vi "测量流程.vi"(11 "控制命令":T1(ring)) -> ()   [LabVIEW 2016, in "斯坦道氟化物.lvlib"]
uses:
  <vilib>/ptbypt/NI_PtbyPt.lvlib
panel:
  out "start":timestamp
  out "重测":bool
  out "x-y":dbl
  out "当前时间":timestamp
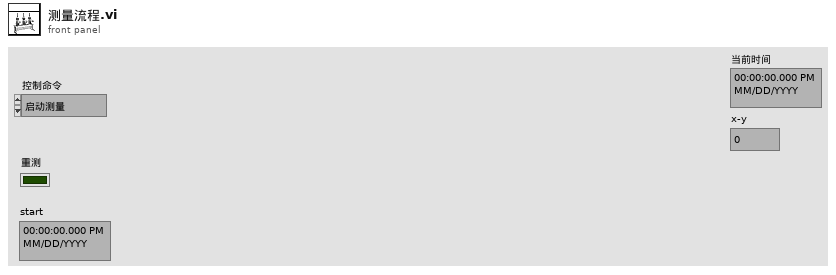
[diagram p1: front panel]
types:
  T1 = enum16{"启动测量", "标样核查", "零点核查", "跨度核查", "空白测试", "平行样测试", "加标回收", "空白校准", "标样校准", "初始化（清洗）", "停止测试", "仪器重启", "校时", "模式设置", "测量间隔设置"}
  T2 = cluster{"时间标识":timestamp, "设备":string, "日志信息":string, "流程参数":string}
  T3 = cluster{"站号":u16, "量程切换":enum32{"H", "L", "AUTO"}, "控制命令":enum16{"启动测量", "标样核查", "零点核查", "跨度核查", "空白测试", "平行样测试", "加标回收", "空白校准", "标样校准", "初始化（清洗）", "停止测试", "仪器重启", "校时", "模式设置", "测量间隔设置"}, "模式设置":enum16{"待机", "连续模式", "周期模式", "定点模式", "受控模式", "手动模式"}, "测量间隔":u16}
  T4 = typedef "报警信息字段定义.ctl" = cluster{"时间":timestamp, "参数":string, "报警信息":string, "备注":string, "code":u64}
  T5 = enum16{"空闲", "水样测试", "标样核查", "零点核查", "跨度核查", "空白测试", "平行样测试", "加标回收", "空白校准", "标样校准", "初始化（清洗）"}
  T6 = cluster{"因子编码":u32, "单位":u16, "标样参考值":sgl, "水样数据时间":timestamp, "水样实测值":sgl, "水样数据标识":string, "标样数据时间":timestamp, "标样实测值":sgl, "标样数据标识":string, "空白数据时间":timestamp, "空白实测值":sgl, "空白数据标识":string, "零点核查数据时间":timestamp, "零点核查实测值":sgl, "零点核查数据标识":string, "跨度核查数据时间":timestamp, "跨度核查实测值":sgl, "跨度核查数据标识":string, "加标回收数据时间":timestamp, "加标回收实测值":sgl, "加标回收数据标识":string, "平行样数据时间":timestamp, "平行样实测值":sgl, "平行样数据标识":string, "F0":sgl, "F1":sgl, "F2":sgl, "F3":sgl, "F4":sgl, "F5":sgl, "F6":sgl, "F7":sgl, "温度":sgl, "湿度":sgl, "X值":sgl, "fidrange":u16, "X1值":sgl}[]
  T7 = cluster{"因子编码":u32, "单位":u16, "标样参考值":sgl, "水样数据时间":timestamp, "水样实测值":sgl, "水样数据标识":string, "标样数据时间":timestamp, "标样实测值":sgl, "标样数据标识":string, "空白数据时间":timestamp, "空白实测值":sgl, "空白数据标识":string, "零点核查数据时间":timestamp, "零点核查实测值":sgl, "零点核查数据标识":string, "跨度核查数据时间":timestamp, "跨度核查实测值":sgl, "跨度核查数据标识":string, "加标回收数据时间":timestamp, "加标回收实测值":sgl, "加标回收数据标识":string, "平行样数据时间":timestamp, "平行样实测值":sgl, "平行样数据标识":string, "F0":sgl, "F1":sgl, "F2":sgl, "F3":sgl, "F4":sgl, "F5":sgl, "F6":sgl, "F7":sgl, "温度":sgl, "湿度":sgl, "X值":sgl, "fidrange":u16, "X1值":sgl}
  T8 = cluster{"总磷跨度值":dbl, "总磷零点标准液浓度":dbl, "总磷跨度标准液浓度":dbl, "总磷标准液标准浓度":dbl, "总氮跨度值":dbl, "总氮零点标准液浓度":dbl, "总氮跨度标准液浓度":dbl, "总氮标准液标准浓度":dbl, "COD跨度值":dbl, "COD零点标准液浓度":dbl, "COD跨度标准液浓度":dbl, "COD标准液标准浓度":dbl, "氨氮跨度值":dbl, "氨氮零点标准液浓度":dbl, "氨氮跨度标准液浓度":dbl, "氨氮标准液标准浓度":dbl, "磷酸盐跨度值":dbl, "磷酸盐零点标准液浓度":dbl, "磷酸盐跨度标准液浓度":dbl, "磷酸盐标准液标准浓度":dbl, "硝氮跨度值":dbl, "硝氮零点标准液浓度":dbl, "硝氮跨度标准液浓度":dbl, "硝氮标准液标准浓度":dbl, "亚硝氮跨度值":dbl, "亚硝氮零点标准液浓度":dbl, "亚硝氮跨度标准液浓度":dbl, "亚硝氮标准液标准浓度":dbl, "硫化物跨度值":dbl, "硫化物零点标准液浓度":dbl, "硫化物跨度标准液浓度":dbl, "硫化物标准液标准浓度":dbl, "硅酸盐跨度值":dbl, "硅酸盐零点标准液浓度":dbl, "硅酸盐跨度标准液浓度":dbl, "硅酸盐标准液标准浓度":dbl, "总磷零点标准液偏差":dbl, "总磷跨度标准液偏差":dbl, "总磷标准液标准偏差":dbl, "总氮零点标准液偏差":dbl, "总氮跨度标准液偏差":dbl, "总氮标准液标准偏差":dbl, "COD零点标准液偏差":dbl, "COD跨度标准液偏差":dbl, "COD标准液标准偏差":dbl, "氨氮零点标准液偏差":dbl, "氨氮跨度标准液偏差":dbl, "氨氮标准液标准偏差":dbl, "磷酸盐零点标准液偏差":dbl, "磷酸盐跨度标准液偏差":dbl, "磷酸盐标准液标准偏差":dbl, "硝氮零点标准液偏差":dbl, "硝氮跨度标准液偏差":dbl, "硝氮标准液标准偏差":dbl, "亚硝氮零点标准液偏差":dbl, "亚硝氮跨度标准液偏差":dbl, "亚硝氮标准液标准偏差":dbl, "硫化物零点标准液偏差":dbl, "硫化物跨度标准液偏差":dbl, "硫化物标准液标准偏差":dbl, "硅酸盐零点标准液偏差":dbl, "硅酸盐跨度标准液偏差":dbl, "硅酸盐标准液标准偏差":dbl, "氟化物跨度值":dbl, "氟化物零点标准液浓度":dbl, "氟化物跨度标准液浓度":dbl, "氟化物标准液标准浓度":dbl, "氟化物零点标准液偏差":dbl, "氟化物跨度标准液偏差":dbl, "氟化物标准液标准偏差":dbl}
  T9 = cluster{"系统时间":timestamp, "工作状态":u16, "测量模式":enum16{"待机", "连续模式", "周期模式", "定点模式", "受控模式", "手动模式"}, "告警代码":u16, "故障代码":u16, "日志代码":u16, "软件版本":u16, "F0":sgl, "F1":sgl, "F2":sgl, "F3":sgl, "T":sgl, "H":sgl, "id":u16, "flowid":u16, "量程":u16, "总磷控温温度1":sgl, "营养盐控温温度2":sgl, "ADC":sgl}
  T10 = cluster{"水样测试量程模式":enum16{"H", "L", "AUTO"}, "空白核查量程模式":enum16{"H", "L", "AUTO"}, "跨度核查量程模式":enum16{"H", "L", "AUTO"}, "加标回收量程模式":enum16{"H", "L", "AUTO"}, "标样核查量程模式":enum16{"H", "L", "AUTO"}}
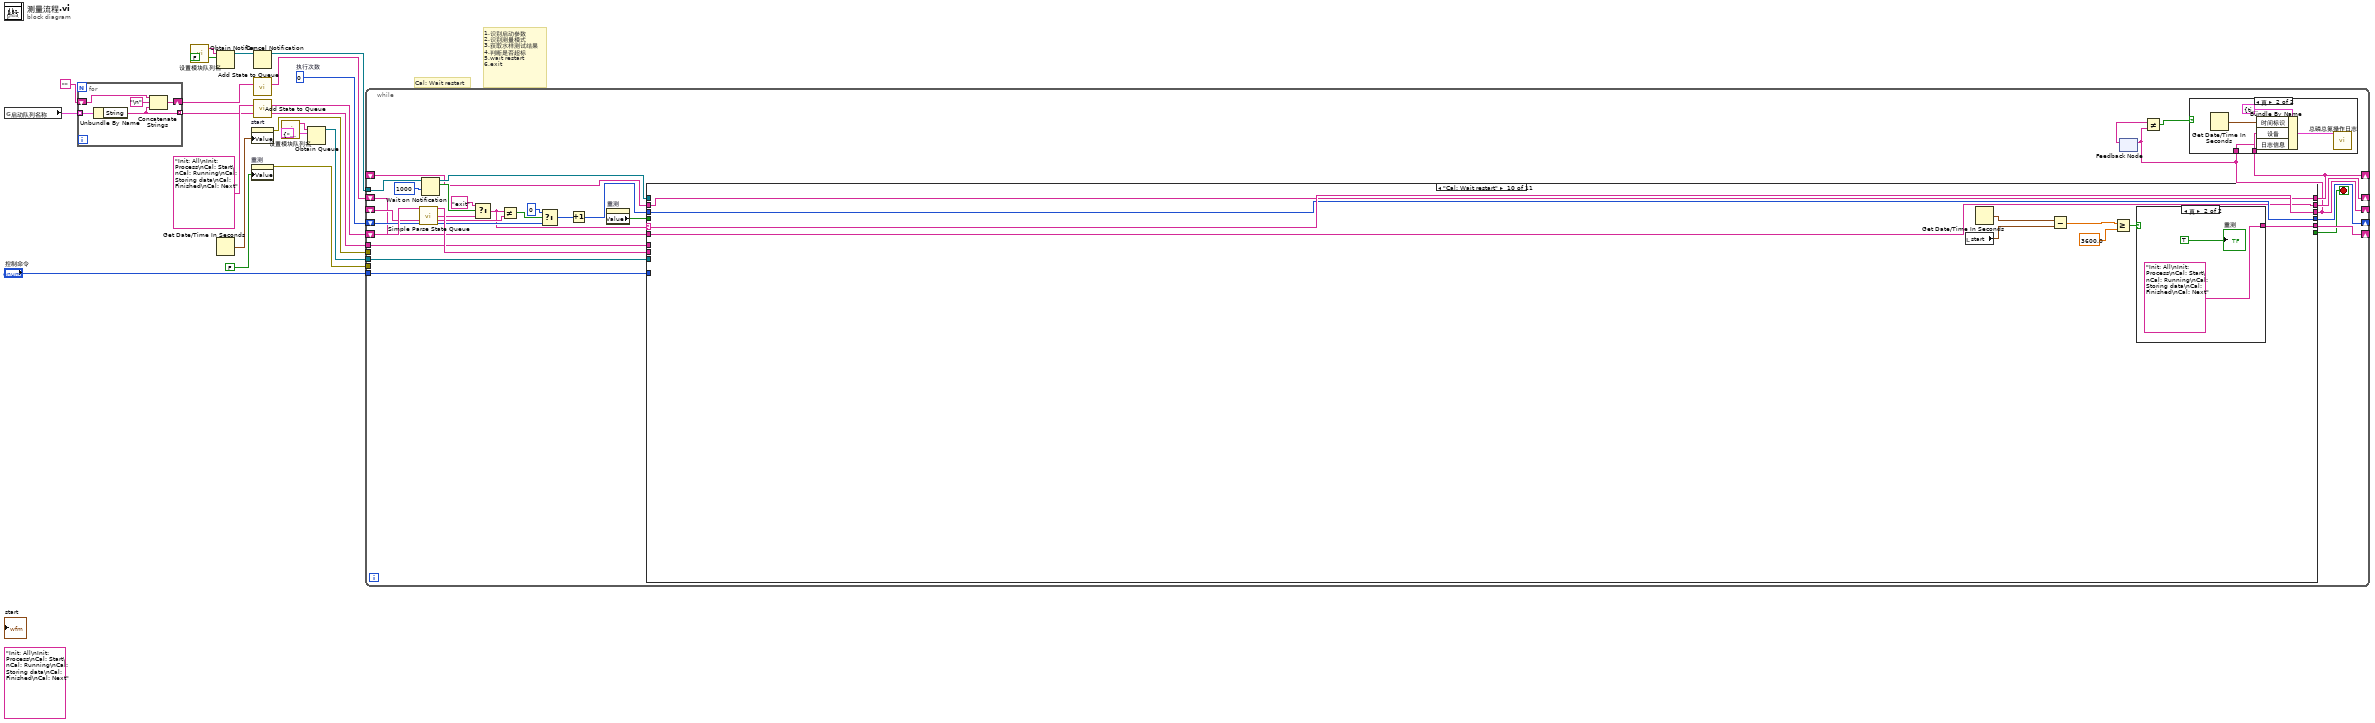
[diagram p0: block diagram]
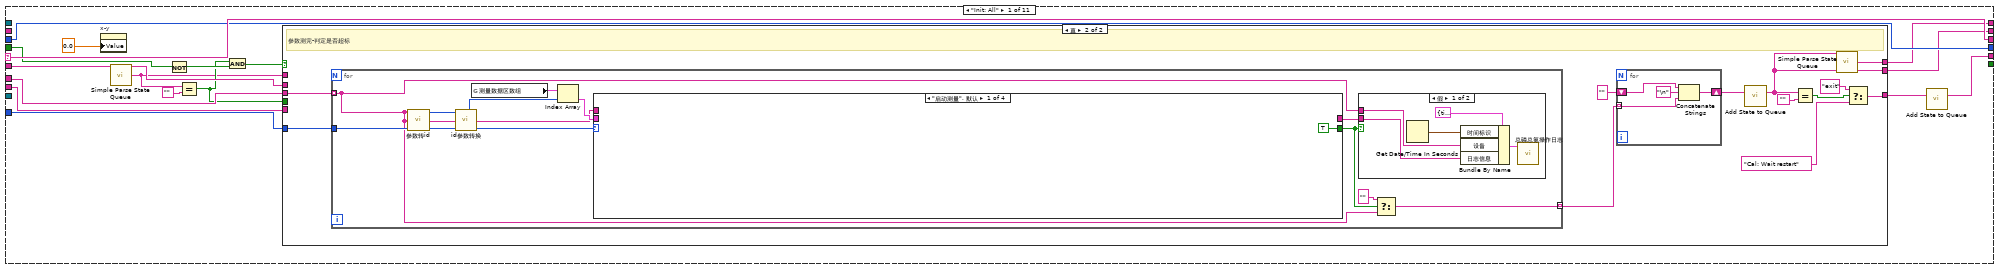
[diagram p3: hidden frame]
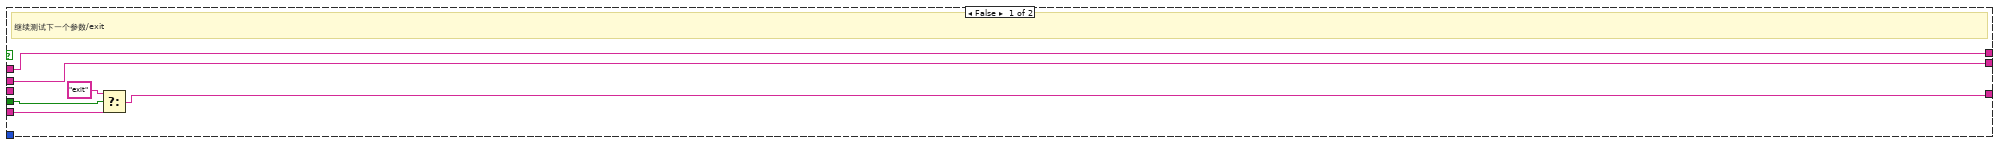
[diagram p4: hidden frame]
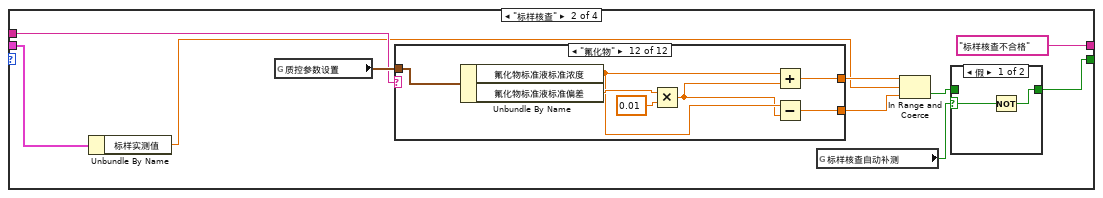
[diagram p6: hidden frame]
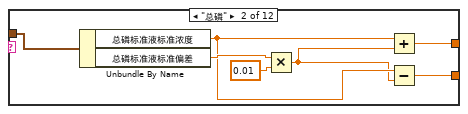
[diagram p9: hidden frame]
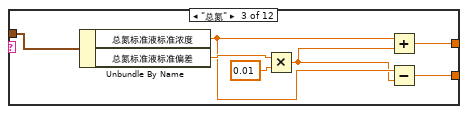
[diagram p10: hidden frame]
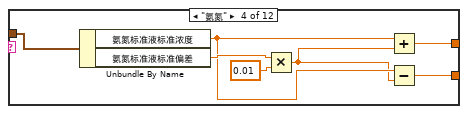
[diagram p11: hidden frame]
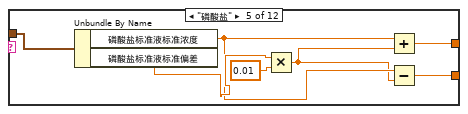
[diagram p12: hidden frame]
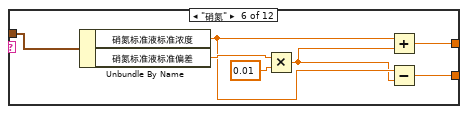
[diagram p13: hidden frame]
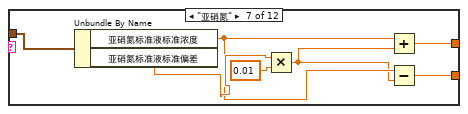
[diagram p14: hidden frame]
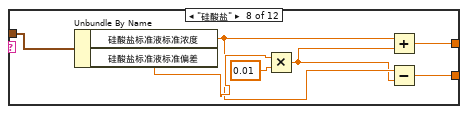
[diagram p15: hidden frame]
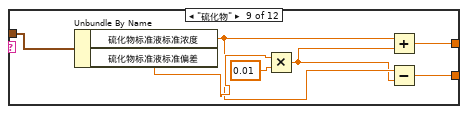
[diagram p16: hidden frame]
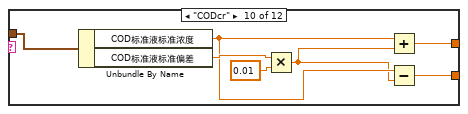
[diagram p17: hidden frame]
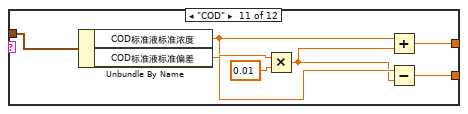
[diagram p18: hidden frame]
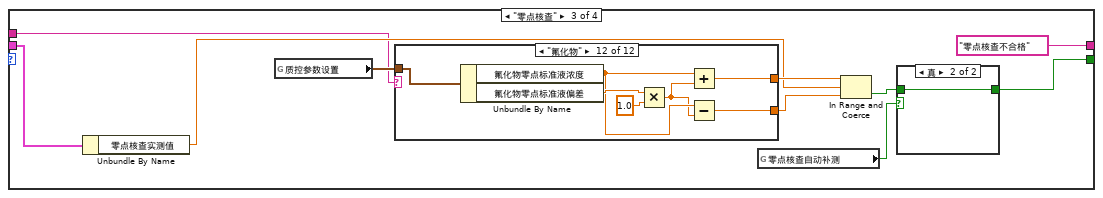
[diagram p19: hidden frame]
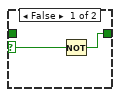
[diagram p20: hidden frame]
diagram:
  (unwired) "Init: All\nInit: Process\nCal: Start\nCal: Running\nCal: Storing data\nCal: Finished\nCal: Next" ("State(s) In (\"\")")
  w14 = 0  # 执行次数
  # "Cal: Wait restart"
  # "1.识别启动参数\n2.识别测量模式\n3.获取水样测试结果\n4.判断是否超标\n5.wait restart\n6.exit"
  n1 = global read "model config var.vi" "启动队列名称"() -> (w7:cluster{"String":string, "Value":u16}[])
  n2 = for {
    shift-right: [w24] -> w8
    shift-left: "" -> [w25]
    tunnel: w7 -> [w23] mode=indexing
    tunnel: [w21] -> w5 mode=indexing
    n3 = Unbundle By Name(w23) -> ("String"=w21:string)
    n4 = Concatenate Strings(w25, "\n", w21) -> (w24:string)
  }
  n5 = call "设置模块队列名.vi"() -> ("Msg"=w12:string)  [unwired: 5 in]
  n6 = Obtain Notifier(name (unnamed)=w12, notification data type=FALSE) -> (notifier out=w19:refnum<notifier>)  [unwired: 2 in, 2 out]
  n7 = Get Date/Time In Seconds() -> (seconds since 1Jan1904=w1:timestamp)
  n8 = property on="start" class="AbsTime (严格)"("Value"=w1) -> (error out=w2:errorcluster)  [unwired: 2 in, 1 out]
  n9 = property on="重测" class="Bool (严格)"("Value"=FALSE ("重测")) -> (error out=w3:errorcluster)  [unwired: 2 in, 1 out]
  n10 = Cancel Notification(0:w19) -> (8:w10:refnum<notifier>)  [unwired: 1 in, 2 out]
  n11 = call "Add State to Queue.vi"("State(s) In (\"\")"=w8) -> ("States Out"=w13:string)  [unwired: 14 in]
  n12 = call "Add State to Queue.vi"("State(s) In (\"\")"="Init: All\nInit: Process\nCal: Start\nCal: Running\nCal: Storing data\nCal: Finished\nCal: Next" ("State(s) In (\"\")")) -> ("States Out"=w17:string)  [unwired: 14 in]
  n13 = call "设置模块队列名.vi"() -> ("Msg"=w11:string)  [unwired: 5 in]
  n14 = Obtain Queue(name (unnamed)=w11, element data type=cluster{"命令":string, "data":variant} {"命令"="", "data"=variant}) -> (queue out=w15:refnum<queue>)  [unwired: 3 in, 2 out]
  n15 = while {
    tunnel: w15 -> [w52]
    shift-right: [w51] -> _
    shift-left: w17 -> [w54]
    shift-right: [w45] -> _
    shift-left: w14 -> [w48]
    shift-right: [w27] -> _
    shift-left: _ -> [w50]
    tunnel: "控制命令" -> [w43]
    shift-right: [w41] -> _
    shift-left: w13 -> [w31]
    shift-right: [w29] -> _
    shift-left: _ -> [w30]
    tunnel: w10 -> [w39]
    tunnel: w5 -> [w33]
    tunnel: w3 -> [_]
    tunnel: w2 -> [_]
    stop <- w42 stop-if-true
    n16 = call "Simple Parse State Queue.vi"("State Queue"=w54) -> ("Remain States"=w53:string, "Next State"=w36:string)  [unwired: 13 in]
    n17 = Wait on Notification(notifier=w39, timeout in ms (-1)=1000 ("超时毫秒(-1)")) -> (notifier out=w34:refnum<notifier>, notification=w38:bool)  [unwired: 2 in, 2 out]
    n18 = Select(t="exit", s=w38, f=w36) -> (s? t:f=w35:string)
    n19 = Not Equal?(x=w35, y=w50) -> (x != y?=w49:bool)
    n20 = Select(t=0, s=w49, f=w48) -> (s? t:f=w46:i32)
    n21 = Increment(x=w46) -> (x+1=w44:i32)
    n22 = property on="重测" class="Bool (严格)"() -> ("Value"=w32:bool)  [unwired: 2 in, 2 out]
    n23 = case shown="\"Cal: Wait restart\"" w35 {
      selector: w35 -> [w76 w394 w434 w495 w510 w516 w530 w547 w561 w572 w585]
      tunnel: w53 -> [w70 w404 w436 w497 _ w527 w535 w549 _ _ w586]
      tunnel: w52 -> [_ _ w432 _ _ _ _ _ _ _ w582]
      tunnel: [w77 w405 w435 w496 w511 w526 w534 w548 "Init: All\nInit: Process\nCal: Start\nCal: Running\nCal: Storing data\nCal: Finished\nCal: Next" ("State(s) In (\"\")") w567 w586] -> w51
      tunnel: [w76 w394 w434 w495 w510 w516 w530 w547 w561 w572 w585] -> w27
      tunnel: [w75 w393 w414 w494 w509 w519 w533 w545 w560 w571 w584] -> w45
      tunnel: w44 -> [w75 w393 w414 w494 w509 w519 w533 w545 w560 w571 w584]
      tunnel: w43 -> [w71 w398 w431 _ _ _ _ _ _ _ _]
      tunnel: [_ _ _ _ _ _ _ _ _ _ TRUE] -> w42
      tunnel: w31 -> [w68 w403 w422 w493 w503 w513 w537 w546 w559 w570 w583]
      tunnel: [w62 w401 w416 w492 w502 w512 w536 w544 w558 w569 w577] -> w29
      tunnel: [w66 w403 w422 w493 w503 w513 w537 w546 w559 w570 w583] -> w41
      tunnel: w30 -> [_ w401 w416 w492 w502 w512 w536 w544 w558 w569 w577]
      tunnel: w34 -> [_ _ _ _ _ _ _ _ _ _ w581]
      tunnel: w33 -> [w72 _ _ _ _ _ _ _ _ _ _]
      tunnel: w32 -> [w60 _ w413 _ _ _ _ w543 _ _ _]
      frame "Init: All" {
        n24 = property on="x-y" class="DigNum (严格)"("Value"=0.0 ("x-y")) -> ()  [unwired: 2 in, 2 out]
        n25 = call "Simple Parse State Queue.vi"("State Queue"=w68) -> ("Remain States"=w67:string, "Next State"=w61:string)  [unwired: 13 in]
        n26 = Not(x=w60) -> (.not. x?=w64:bool)
        n27 = Equal?(x=w61, y="") -> (x = y?=w63:bool)
        n28 = And(x=w63, y=w64) -> (x .and. y?=w65:bool)
        n29 = case shown="真" w65 {
          tunnel: w72 -> [_ w95]
          tunnel: w71 -> [_ w94]
          tunnel: w70 -> [w80 _]
          tunnel: [w79 w88] -> w69
          tunnel: w67 -> [w83 _]
          tunnel: [w83 w84] -> w66
          tunnel: w63 -> [w81 _]
          tunnel: [w78 w85] -> w62
          tunnel: w61 -> [w78 _]
          frame False {
            # "继续测试下一个参数/exit"
            n30 = Select(t="exit", s=w81, f=w80) -> (s? t:f=w79:string)
          }
          frame True {
            # "参数测完-判定是否超标"
            n31 = for {
              tunnel: w95 -> [w101] mode=indexing
              tunnel: w94 -> [w109]
              tunnel: [w103] -> w93 mode=indexing
              n32 = call "参数转id.vi"("table"=w101) -> ("id"=w108:u16)  [unwired: 10 in]
              n33 = call "id参数转换.vi"("id"=w108) -> ("数组资源索引"=w107:i32)  [unwired: 9 in, 1 out]
              n34 = global read "VAR总磷总氮全局变量.vi" "测量数据区数组"() -> (w106:T6)
              n35 = Index Array(array=w106, index=w107) -> (element=w105:T7)
              n36 = case shown="\"启动测量\", 默认" w109 {
                tunnel: w105 -> [_ w125 w210 w301]
                tunnel: w101 -> [_ w121 w211 w300]
                tunnel: [TRUE w116 w206 w296] -> w102
                tunnel: [_ "标样核查不合格" ("日志信息") "零点核查不合格" ("日志信息") "跨度核查不合格" ("日志信息")] -> w100
                frame "启动测量", Default {
                }
                frame "标样核查" {
                  n37 = Unbundle By Name(w125) -> ("标样实测值"=w120:sgl)
                  n38 = global read "总磷总氮断电保存全局变量.vi" "质控参数设置"() -> (w124:T8)
                  n39 = case shown="\"氟化物\"" w121 {
                    tunnel: w124 -> [_ w135 w138 w145 w152 w159 w166 w173 w180 w187 w194 w201]
                    tunnel: [_ w132 w137 w144 w151 w158 w165 w172 w179 w186 w193 w200] -> w123
                    tunnel: [_ w131 w136 w143 w150 w157 w164 w171 w178 w185 w192 w199] -> w122
                    frame Default {
                    }
                    frame "总磷" {
                      n40 = Unbundle By Name(w135) -> ("总磷标准液标准浓度"=w130:dbl, "总磷标准液标准偏差"=w134:dbl)
                      n41 = Multiply(x=w134, y=0.01) -> (x*y=w129:dbl)
                      n42 = Add(x=w130, y=w129) -> (x+y=w132:dbl)
                      n43 = Subtract(x=w130, y=w129) -> (x-y=w131:dbl)
                    }
                    frame "总氮" {
                      n44 = Unbundle By Name(w138) -> ("总氮标准液标准浓度"=w140:dbl, "总氮标准液标准偏差"=w142:dbl)
                      n45 = Multiply(x=w142, y=0.01) -> (x*y=w139:dbl)
                      n46 = Add(x=w140, y=w139) -> (x+y=w137:dbl)
                      n47 = Subtract(x=w140, y=w139) -> (x-y=w136:dbl)
                    }
                    frame "氨氮" {
                      n48 = Unbundle By Name(w145) -> ("氨氮标准液标准浓度"=w147:dbl, "氨氮标准液标准偏差"=w149:dbl)
                      n49 = Multiply(x=w149, y=0.01) -> (x*y=w146:dbl)
                      n50 = Add(x=w147, y=w146) -> (x+y=w144:dbl)
                      n51 = Subtract(x=w147, y=w146) -> (x-y=w143:dbl)
                    }
                    frame "磷酸盐" {
                      n52 = Unbundle By Name(w152) -> ("磷酸盐标准液标准浓度"=w154:dbl, "磷酸盐标准液标准偏差"=w156:dbl)
                      n53 = Multiply(x=w156, y=0.01) -> (x*y=w153:dbl)
                      n54 = Add(x=w154, y=w153) -> (x+y=w151:dbl)
                      n55 = Subtract(x=w154, y=w153) -> (x-y=w150:dbl)
                    }
                    frame "硝氮" {
                      n56 = Unbundle By Name(w159) -> ("硝氮标准液标准浓度"=w161:dbl, "硝氮标准液标准偏差"=w163:dbl)
                      n57 = Multiply(x=w163, y=0.01) -> (x*y=w160:dbl)
                      n58 = Add(x=w161, y=w160) -> (x+y=w158:dbl)
                      n59 = Subtract(x=w161, y=w160) -> (x-y=w157:dbl)
                    }
                    frame "亚硝氮" {
                      n60 = Unbundle By Name(w166) -> ("亚硝氮标准液标准浓度"=w168:dbl, "亚硝氮标准液标准偏差"=w170:dbl)
                      n61 = Multiply(x=w170, y=0.01) -> (x*y=w167:dbl)
                      n62 = Add(x=w168, y=w167) -> (x+y=w165:dbl)
                      n63 = Subtract(x=w168, y=w167) -> (x-y=w164:dbl)
                    }
                    frame "硅酸盐" {
                      n64 = Unbundle By Name(w173) -> ("硅酸盐标准液标准浓度"=w175:dbl, "硅酸盐标准液标准偏差"=w177:dbl)
                      n65 = Multiply(x=w177, y=0.01) -> (x*y=w174:dbl)
                      n66 = Add(x=w175, y=w174) -> (x+y=w172:dbl)
                      n67 = Subtract(x=w175, y=w174) -> (x-y=w171:dbl)
                    }
                    frame "硫化物" {
                      n68 = Unbundle By Name(w180) -> ("硫化物标准液标准浓度"=w182:dbl, "硫化物标准液标准偏差"=w184:dbl)
                      n69 = Multiply(x=w184, y=0.01) -> (x*y=w181:dbl)
                      n70 = Add(x=w182, y=w181) -> (x+y=w179:dbl)
                      n71 = Subtract(x=w182, y=w181) -> (x-y=w178:dbl)
                    }
                    frame "CODcr" {
                      n72 = Unbundle By Name(w187) -> ("COD标准液标准浓度"=w189:dbl, "COD标准液标准偏差"=w191:dbl)
                      n73 = Multiply(x=w191, y=0.01) -> (x*y=w188:dbl)
                      n74 = Add(x=w189, y=w188) -> (x+y=w186:dbl)
                      n75 = Subtract(x=w189, y=w188) -> (x-y=w185:dbl)
                    }
                    frame "COD" {
                      n76 = Unbundle By Name(w194) -> ("COD标准液标准浓度"=w196:dbl, "COD标准液标准偏差"=w198:dbl)
                      n77 = Multiply(x=w198, y=0.01) -> (x*y=w195:dbl)
                      n78 = Add(x=w196, y=w195) -> (x+y=w193:dbl)
                      n79 = Subtract(x=w196, y=w195) -> (x-y=w192:dbl)
                    }
                    frame "氟化物" {
                      n80 = Unbundle By Name(w201) -> ("氟化物标准液标准浓度"=w203:dbl, "氟化物标准液标准偏差"=w205:dbl)
                      n81 = Multiply(x=w205, y=0.01) -> (x*y=w202:dbl)
                      n82 = Add(x=w203, y=w202) -> (x+y=w200:dbl)
                      n83 = Subtract(x=w203, y=w202) -> (x-y=w199:dbl)
                    }
                  }
                  n84 = global read "总磷总氮断电保存全局变量.vi" "标样核查自动补测"() -> (w118:bool)
                  n85 = In Range and Coerce(upper limit=w123, x=w120, lower limit=w122) -> (In Range?=w117:bool)  [unwired: 1 out]
                  n86 = case shown="假" w118 {
                    selector: w118 -> [w127 _]
                    tunnel: w117 -> [_ w128]
                    tunnel: [w126 w128] -> w116
                    frame False {
                      n87 = Not(x=w127) -> (.not. x?=w126:bool)
                    }
                    frame True {
                    }
                  }
                }
                frame "零点核查" {
                  n88 = Unbundle By Name(w210) -> ("零点核查实测值"=w212:sgl)
                  n89 = global read "总磷总氮断电保存全局变量.vi" "质控参数设置"() -> (w215:T8)
                  n90 = case shown="\"氟化物\"" w211 {
                    tunnel: w215 -> [_ w225 w228 w235 w242 w249 w256 w263 w270 w277 w284 w291]
                    tunnel: [_ w222 w227 w234 w241 w248 w255 w262 w269 w276 w283 w290] -> w214
                    tunnel: [_ w221 w226 w233 w240 w247 w254 w261 w268 w275 w282 w289] -> w213
                    frame Default {
                    }
                    frame "总磷" {
                      n91 = Unbundle By Name(w225) -> ("总磷零点标准液浓度"=w220:dbl, "总磷零点标准液偏差"=w224:dbl)
                      n92 = Multiply(x=w224, y=1.0) -> (x*y=w219:dbl)
                      n93 = Add(x=w220, y=w219) -> (x+y=w222:dbl)
                      n94 = Subtract(x=w220, y=w219) -> (x-y=w221:dbl)
                    }
                    frame "总氮" {
                      n95 = Unbundle By Name(w228) -> ("总氮零点标准液浓度"=w230:dbl, "总氮零点标准液偏差"=w232:dbl)
                      n96 = Multiply(x=w232, y=1.0) -> (x*y=w229:dbl)
                      n97 = Add(x=w230, y=w229) -> (x+y=w227:dbl)
                      n98 = Subtract(x=w230, y=w229) -> (x-y=w226:dbl)
                    }
                    frame "氨氮" {
                      n99 = Unbundle By Name(w235) -> ("氨氮零点标准液浓度"=w237:dbl, "氨氮零点标准液偏差"=w239:dbl)
                      n100 = Multiply(x=w239, y=1.0) -> (x*y=w236:dbl)
                      n101 = Add(x=w237, y=w236) -> (x+y=w234:dbl)
                      n102 = Subtract(x=w237, y=w236) -> (x-y=w233:dbl)
                    }
                    frame "磷酸盐" {
                      n103 = Unbundle By Name(w242) -> ("磷酸盐零点标准液浓度"=w244:dbl, "磷酸盐零点标准液偏差"=w246:dbl)
                      n104 = Multiply(x=w246, y=1.0) -> (x*y=w243:dbl)
                      n105 = Add(x=w244, y=w243) -> (x+y=w241:dbl)
                      n106 = Subtract(x=w244, y=w243) -> (x-y=w240:dbl)
                    }
                    frame "硝氮" {
                      n107 = Unbundle By Name(w249) -> ("硝氮零点标准液浓度"=w251:dbl, "硝氮零点标准液偏差"=w253:dbl)
                      n108 = Multiply(x=w253, y=1.0) -> (x*y=w250:dbl)
                      n109 = Add(x=w251, y=w250) -> (x+y=w248:dbl)
                      n110 = Subtract(x=w251, y=w250) -> (x-y=w247:dbl)
                    }
                    frame "亚硝氮" {
                      n111 = Unbundle By Name(w256) -> ("亚硝氮零点标准液浓度"=w258:dbl, "亚硝氮零点标准液偏差"=w260:dbl)
                      n112 = Multiply(x=w260, y=1.0) -> (x*y=w257:dbl)
                      n113 = Add(x=w258, y=w257) -> (x+y=w255:dbl)
                      n114 = Subtract(x=w258, y=w257) -> (x-y=w254:dbl)
                    }
                    frame "硅酸盐" {
                      n115 = Unbundle By Name(w263) -> ("硅酸盐零点标准液浓度"=w265:dbl, "硅酸盐零点标准液偏差"=w267:dbl)
                      n116 = Multiply(x=w267, y=1.0) -> (x*y=w264:dbl)
                      n117 = Add(x=w265, y=w264) -> (x+y=w262:dbl)
                      n118 = Subtract(x=w265, y=w264) -> (x-y=w261:dbl)
                    }
                    frame "硫化物" {
                      n119 = Unbundle By Name(w270) -> ("硫化物零点标准液浓度"=w272:dbl, "硫化物零点标准液偏差"=w274:dbl)
                      n120 = Multiply(x=w274, y=1.0) -> (x*y=w271:dbl)
                      n121 = Add(x=w272, y=w271) -> (x+y=w269:dbl)
                      n122 = Subtract(x=w272, y=w271) -> (x-y=w268:dbl)
                    }
                    frame "CODcr" {
                      n123 = Unbundle By Name(w277) -> ("COD零点标准液浓度"=w279:dbl, "COD零点标准液偏差"=w281:dbl)
                      n124 = Multiply(x=w281, y=1.0) -> (x*y=w278:dbl)
                      n125 = Add(x=w279, y=w278) -> (x+y=w276:dbl)
                      n126 = Subtract(x=w279, y=w278) -> (x-y=w275:dbl)
                    }
                    frame "COD" {
                      n127 = Unbundle By Name(w284) -> ("COD零点标准液浓度"=w286:dbl, "COD零点标准液偏差"=w288:dbl)
                      n128 = Multiply(x=w288, y=1.0) -> (x*y=w285:dbl)
                      n129 = Add(x=w286, y=w285) -> (x+y=w283:dbl)
                      n130 = Subtract(x=w286, y=w285) -> (x-y=w282:dbl)
                    }
                    frame "氟化物" {
                      n131 = Unbundle By Name(w291) -> ("氟化物零点标准液浓度"=w293:dbl, "氟化物零点标准液偏差"=w295:dbl)
                      n132 = Multiply(x=w295, y=1.0) -> (x*y=w292:dbl)
                      n133 = Add(x=w293, y=w292) -> (x+y=w290:dbl)
                      n134 = Subtract(x=w293, y=w292) -> (x-y=w289:dbl)
                    }
                  }
                  n135 = global read "总磷总氮断电保存全局变量.vi" "零点核查自动补测"() -> (w208:bool)
                  n136 = In Range and Coerce(upper limit=w214, x=w212, lower limit=w213) -> (In Range?=w207:bool)  [unwired: 1 out]
                  n137 = case shown="真" w208 {
                    selector: w208 -> [w217 _]
                    tunnel: w207 -> [_ w218]
                    tunnel: [w216 w218] -> w206
                    frame False {
                      n138 = Not(x=w217) -> (.not. x?=w216:bool)
                    }
                    frame True {
                    }
                  }
                }
                frame "跨度核查" {
                  n139 = Unbundle By Name(w301) -> ("跨度核查实测值"=w302:sgl)
                  n140 = global read "总磷总氮断电保存全局变量.vi" "质控参数设置"() -> (w305:T8)
                  n141 = case shown="\"氟化物\"" w300 {
                    tunnel: w305 -> [_ w315 w318 w325 w332 w339 w346 w353 w360 w367 w374 w381]
                    tunnel: [_ w312 w317 w324 w331 w338 w345 w352 w359 w366 w373 w380] -> w304
                    tunnel: [_ w311 w316 w323 w330 w337 w344 w351 w358 w365 w372 w379] -> w303
                    frame Default {
                    }
                    frame "总磷" {
                      n142 = Unbundle By Name(w315) -> ("总磷跨度标准液浓度"=w310:dbl, "总磷跨度标准液偏差"=w314:dbl)
                      n143 = Multiply(x=w314, y=0.01) -> (x*y=w309:dbl)
                      n144 = Add(x=w310, y=w309) -> (x+y=w312:dbl)
                      n145 = Subtract(x=w310, y=w309) -> (x-y=w311:dbl)
                    }
                    frame "总氮" {
                      n146 = Unbundle By Name(w318) -> ("总氮跨度标准液浓度"=w320:dbl, "总氮跨度标准液偏差"=w322:dbl)
                      n147 = Multiply(x=w322, y=0.01) -> (x*y=w319:dbl)
                      n148 = Add(x=w320, y=w319) -> (x+y=w317:dbl)
                      n149 = Subtract(x=w320, y=w319) -> (x-y=w316:dbl)
                    }
                    frame "氨氮" {
                      n150 = Unbundle By Name(w325) -> ("氨氮跨度标准液浓度"=w327:dbl, "氨氮跨度标准液偏差"=w329:dbl)
                      n151 = Multiply(x=w329, y=0.01) -> (x*y=w326:dbl)
                      n152 = Add(x=w327, y=w326) -> (x+y=w324:dbl)
                      n153 = Subtract(x=w327, y=w326) -> (x-y=w323:dbl)
                    }
                    frame "磷酸盐" {
                      n154 = Unbundle By Name(w332) -> ("磷酸盐跨度标准液浓度"=w334:dbl, "磷酸盐跨度标准液偏差"=w336:dbl)
                      n155 = Multiply(x=w336, y=0.01) -> (x*y=w333:dbl)
                      n156 = Add(x=w334, y=w333) -> (x+y=w331:dbl)
                      n157 = Subtract(x=w334, y=w333) -> (x-y=w330:dbl)
                    }
                    frame "硝氮" {
                      n158 = Unbundle By Name(w339) -> ("硝氮跨度标准液浓度"=w341:dbl, "硝氮跨度标准液偏差"=w343:dbl)
                      n159 = Multiply(x=w343, y=0.01) -> (x*y=w340:dbl)
                      n160 = Add(x=w341, y=w340) -> (x+y=w338:dbl)
                      n161 = Subtract(x=w341, y=w340) -> (x-y=w337:dbl)
                    }
                    frame "亚硝氮" {
                      n162 = Unbundle By Name(w346) -> ("亚硝氮跨度标准液浓度"=w348:dbl, "亚硝氮跨度标准液偏差"=w350:dbl)
                      n163 = Multiply(x=w350, y=0.01) -> (x*y=w347:dbl)
                      n164 = Add(x=w348, y=w347) -> (x+y=w345:dbl)
                      n165 = Subtract(x=w348, y=w347) -> (x-y=w344:dbl)
                    }
                    frame "硅酸盐" {
                      n166 = Unbundle By Name(w353) -> ("硅酸盐跨度标准液浓度"=w355:dbl, "硅酸盐跨度标准液偏差"=w357:dbl)
                      n167 = Multiply(x=w357, y=0.01) -> (x*y=w354:dbl)
                      n168 = Add(x=w355, y=w354) -> (x+y=w352:dbl)
                      n169 = Subtract(x=w355, y=w354) -> (x-y=w351:dbl)
                    }
                    frame "硫化物" {
                      n170 = Unbundle By Name(w360) -> ("硫化物跨度标准液浓度"=w362:dbl, "硫化物跨度标准液偏差"=w364:dbl)
                      n171 = Multiply(x=w364, y=0.01) -> (x*y=w361:dbl)
                      n172 = Add(x=w362, y=w361) -> (x+y=w359:dbl)
                      n173 = Subtract(x=w362, y=w361) -> (x-y=w358:dbl)
                    }
                    frame "CODcr" {
                      n174 = Unbundle By Name(w367) -> ("COD跨度标准液浓度"=w369:dbl, "COD跨度标准液偏差"=w371:dbl)
                      n175 = Multiply(x=w371, y=0.01) -> (x*y=w368:dbl)
                      n176 = Add(x=w369, y=w368) -> (x+y=w366:dbl)
                      n177 = Subtract(x=w369, y=w368) -> (x-y=w365:dbl)
                    }
                    frame "COD" {
                      n178 = Unbundle By Name(w374) -> ("COD跨度标准液浓度"=w376:dbl, "COD跨度标准液偏差"=w378:dbl)
                      n179 = Multiply(x=w378, y=0.01) -> (x*y=w375:dbl)
                      n180 = Add(x=w376, y=w375) -> (x+y=w373:dbl)
                      n181 = Subtract(x=w376, y=w375) -> (x-y=w372:dbl)
                    }
                    frame "氟化物" {
                      n182 = Unbundle By Name(w381) -> ("氟化物跨度标准液浓度"=w383:dbl, "氟化物跨度标准液偏差"=w385:dbl)
                      n183 = Multiply(x=w385, y=0.01) -> (x*y=w382:dbl)
                      n184 = Add(x=w383, y=w382) -> (x+y=w380:dbl)
                      n185 = Subtract(x=w383, y=w382) -> (x-y=w379:dbl)
                    }
                  }
                  n186 = global read "总磷总氮断电保存全局变量.vi" "跨度核查自动补测"() -> (w298:bool)
                  n187 = In Range and Coerce(upper limit=w304, x=w302, lower limit=w303) -> (In Range?=w297:bool)  [unwired: 1 out]
                  n188 = case shown="真" w298 {
                    selector: w298 -> [w307 _]
                    tunnel: w297 -> [_ w308]
                    tunnel: [w306 w308] -> w296
                    frame False {
                      n189 = Not(x=w307) -> (.not. x?=w306:bool)
                    }
                    frame True {
                    }
                  }
                }
              }
              n190 = case shown="假" w102 {
                tunnel: w101 -> [w111 _]
                tunnel: w100 -> [w110 _]
                frame False {
                  n191 = Get Date/Time In Seconds() -> (seconds since 1Jan1904=w114:timestamp)
                  n192 = Bundle By Name(cluster=T2 {"时间标识"=timestamp(0 s since 1904-01-01), "设备"="", "日志信息"="", "流程参数"=""} ("data in"), "时间标识"=w114, "设备"=w111, "日志信息"=w110) -> (w113:T2)
                  n193 = call "总磷总氮操作日志.vi"("data in"=w113) -> ()  [unwired: 10 in, 1 out]
                }
                frame True {
                }
              }
              n194 = Select(t="", s=w102, f=w101) -> (s? t:f=w103:string)
            }
            n195 = for {
              shift-right: [w98] -> w91
              shift-left: "" -> [w99]
              tunnel: w93 -> [w96] mode=indexing
              n196 = Concatenate Strings(w99, "\n", w96) -> (w98:string)
            }
            n197 = call "Add State to Queue.vi"("State(s) In (\"\")"=w91) -> ("States Out"=w84:string)  [unwired: 14 in]
            n198 = Equal?(x=w84, y="") -> (x = y?=w89:bool)
            n199 = call "Simple Parse State Queue.vi"("State Queue"=w84) -> ("Next State"=w85:string)  [unwired: 13 in, 1 out]
            n200 = Select(t="exit", s=w89, f="Cal: Wait restart") -> (s? t:f=w88:string)
          }
        }
        n201 = call "Add State to Queue.vi"("State(s) In (\"\")"=w69) -> ("States Out"=w77:string)  [unwired: 14 in]
      }
      frame "Init: Process" {
        n202 = global read "VAR总磷总氮全局变量.vi" "状态告警区"() -> (w402:T9)
        n203 = call "参数转id.vi"("table"=w401) -> ("id"=w399:u16)  [unwired: 10 in]
        n204 = Greater Or Equal?(x=w393, y=7200) -> (x >= y?=w391:bool)
        n205 = Unbundle By Name(w402) -> ("id"=w400:u16, "工作状态"=w396:u16)
        n206 = Equal?(x=w399, y=w400) -> (x = y?=w387:bool)
        n207 = Not Equal To 0?(x=w396) -> (x != 0?=w397:bool)
        n208 = case shown="真" w397 {
          tunnel: w396 -> [_ w412]
          tunnel: w398 -> [_ w410]
          tunnel: [TRUE w407] -> w386
          tunnel: w387 -> [_ w408]
          frame False {
          }
          frame True {
            n209 = Decrement(x=w412) -> (x-1=w411:u16)
            n210 = Equal?(x=w411, y=w410) -> (x = y?=w409:bool)
            n211 = And(x=w408, y=w409) -> (x .and. y?=w407:bool)
          }
        }
        n212 = Select(t="", s=w386, f=w394) -> (s? t:f=w389:string)
        n213 = Select(t="Cal: Failure", s=w391, f=w389) -> (s? t:f=w388:string)
        n214 = call "Add State to Queue.vi"("State(s) In Front (\"\")"=w388, "State(s) In (\"\")"=w404) -> ("States Out"=w405:string)  [unwired: 13 in]
      }
      frame "Cal: Start" {
        n215 = global read "VAR总磷总氮全局变量.vi" "状态告警区"() -> (w433:T9)
        n216 = case shown="1" w414 {
          tunnel: w416 -> [_ w485]
          tunnel: w413 -> [_ w484]
          frame 0, Default {
          }
          frame 1 {
            n217 = case shown="真" w484 {
              tunnel: [">>开始测量" ("日志信息") ">>开始补测" ("日志信息")] -> w486
              frame False {
              }
              frame True {
              }
            }
            n218 = Get Date/Time In Seconds() -> (seconds since 1Jan1904=w489:timestamp)
            n219 = Bundle By Name(cluster=T2 {"时间标识"=timestamp(0 s since 1904-01-01), "设备"="", "日志信息"="", "流程参数"=""} ("data in"), "时间标识"=w489, "设备"=w485, "日志信息"=w486) -> (w488:T2)
            n220 = call "总磷总氮操作日志.vi"("data in"=w488) -> ()  [unwired: 10 in, 1 out]
          }
        }
        n221 = call "参数转id.vi"("table"=w416) -> ("id"=w415:u16)  [unwired: 10 in]
        n222 = Unbundle By Name(w433) -> ("工作状态"=w421:u16)
        n223 = Equal?(x=w421, y=u16 0) -> (x = y?=w419:bool)
        n224 = call <vilib>:"Boolean Crossing PtByPt.vi"("direction"=enum16{"either", "false-true", "true-false"}."false-true", "input"=w419) -> ("crossing"=w417:bool)  [unwired: 1 in]
        n225 = case shown="真" w419 {
          tunnel: w431 -> [_ w458]
          tunnel: w432 -> [_ w461]
          tunnel: [w441 _] -> w426
          tunnel: w415 -> [_ w456]
          tunnel: w414 -> [_ _]
          tunnel: w416 -> [_ w450]
          tunnel: w417 -> [_ w448]
          frame False {
            n226 = global read "VAR总磷总氮全局变量.vi" "状态告警区"() -> (w440:T9)
            n227 = Unbundle By Name(w440) -> ("故障代码"=w438:u16, "告警代码"=w439:u16)
            n228 = Add(x=w438, y=w439) -> (x+y=w437:u16)
            n229 = case shown="0" w437 {
              tunnel: [w442 TRUE] -> w441
              frame 0 {
                n230 = local read "当前时间"() -> (w446:timestamp)
                n231 = Get Date/Time In Seconds() -> (seconds since 1Jan1904=w445:timestamp)
                n232 = Subtract(x=w445, y=w446) -> (x-y=w444:dbl)
                "x-y" <- w444
                n233 = Greater Or Equal?(x=w444, y=90.0) -> (x >= y?=w442:bool)
              }
              frame 1, Default {
              }
            }
          }
          frame True {
            n234 = property on="x-y" class="DigNum (严格)"() -> ("Value"=w452:dbl)  [unwired: 2 in, 2 out]
            n235 = case shown="50" w456 {
              tunnel: [_ w468 w469 w470 w471 w472 w473 w474 w475 w476 w477] -> w457
              frame 0, Default {
              }
              frame 1 {
                n236 = global read "总磷总氮断电保存全局变量.vi" "总磷自动测试量程配置"() -> (w468:T10)
              }
              frame 2 {
                n237 = global read "总磷总氮断电保存全局变量.vi" "总氮自动测试量程配置"() -> (w469:T10)
              }
              frame 3 {
                n238 = global read "总磷总氮断电保存全局变量.vi" "氨氮自动测试量程配置"() -> (w470:T10)
              }
              frame 4 {
                n239 = global read "总磷总氮断电保存全局变量.vi" "磷酸盐自动测试量程配置"() -> (w471:T10)
              }
              frame 5 {
                n240 = global read "总磷总氮断电保存全局变量.vi" "硝氮自动测试量程配置"() -> (w472:T10)
              }
              frame 6 {
                n241 = global read "总磷总氮断电保存全局变量.vi" "亚硝氮自动测试量程配置"() -> (w473:T10)
              }
              frame 7 {
                n242 = global read "总磷总氮断电保存全局变量.vi" "硅酸盐自动测试量程配置"() -> (w474:T10)
              }
              frame 8 {
                n243 = global read "总磷总氮断电保存全局变量.vi" "硫化物自动测试量程配置"() -> (w475:T10)
              }
              frame 22 {
                n244 = global read "总磷总氮断电保存全局变量.vi" "COD自动测试量程配置"() -> (w476:T10)
              }
              frame 50 {
                n245 = global read "总磷总氮断电保存全局变量.vi" "氟化物自动测试量程配置"() -> (w477:T10)
              }
            }
            n246 = Get Date/Time In Seconds() -> (seconds since 1Jan1904=→"当前时间":timestamp)
            n247 = Not Equal To 0?(x=w452) -> (x != 0?=w451:bool)
            n248 = And(x=w451, y=w448) -> (x .and. y?=w449:bool)
            n249 = case shown="真" w449 {
              tunnel: w450 -> [_ w465]
              frame False {
              }
              frame True {
                n250 = Get Date/Time In Seconds() -> (seconds since 1Jan1904=w464:timestamp)
                n251 = Bundle By Name(cluster=T4 {"时间"=timestamp(0 s since 1904-01-01), "参数"="", "报警信息"="", "备注"="", "code"=0} ("data in"), "时间"=w464, "参数"=w465, "报警信息"="启动失败，正在尝试重新启动") -> (w466:T4)
                n252 = call "总磷总氮报警信息.vi"("data in"=w466) -> ()  [unwired: 10 in, 1 out]
              }
            }
            n253 = Flush Queue(queue=w461) -> (queue out=w454:refnum<queue>)  [unwired: 1 in, 2 out]
            n254 = case shown="\"启动测量\", 默认" w458 {
              tunnel: w457 -> [w479 w481 w483]
              tunnel: [w478 w480 w482] -> w462
              frame "启动测量", Default {
                n255 = Unbundle By Name(w479) -> ("水样测试量程模式"=w478:enum16{"H", "L", "AUTO"})
              }
              frame "零点核查", "空白测试", "空白校准" {
                n256 = Unbundle By Name(w481) -> ("空白核查量程模式"=w480:enum16{"H", "L", "AUTO"})
              }
              frame "标样核查", "跨度核查", "标样校准" {
                n257 = Unbundle By Name(w483) -> ("跨度核查量程模式"=w482:enum16{"H", "L", "AUTO"})
              }
            }
            n258 = Bundle By Name(cluster=T3 {"站号"=1, "量程切换"=enum."AUTO", "控制命令"=enum."启动测量", "模式设置"=enum."待机", "测量间隔"=0} ("参数"), "站号"=w456, "量程切换"=w462, "控制命令"=w458) -> (w459:T3)
            n259 = call "总磷总氮启动命令.vi"("参数"=w459) -> ("启动命令"=w455:cluster{"命令":string, "data":variant})  [unwired: 10 in]
            n260 = Enqueue Element At Opposite End(queue=w454, element=w455) -> ()  [unwired: 2 in, 3 out]
          }
        }
        n261 = Greater Or Equal?(x=w414, y=180) -> (x >= y?=w429:bool)
        n262 = Select(t="Cal: Success" ("State(s) In (\"\")"), s=w426, f="Cal: Start" ("State(s) In (\"\")")) -> (s? t:f=w424:string)
        n263 = Select(t="Cal: Failure" ("State(s) In (\"\")"), s=w429, f=w424) -> (s? t:f=w427:string)
        n264 = call "Add State to Queue.vi"("State(s) In Front (\"\")"=w427, "State(s) In (\"\")"=w436) -> ("States Out"=w435:string)  [unwired: 13 in]
      }
      frame "Cal: Success" {
        n265 = Get Date/Time In Seconds() -> (seconds since 1Jan1904=w500:timestamp)
        n266 = Bundle By Name(cluster=T2 {"时间标识"=timestamp(0 s since 1904-01-01), "设备"="", "日志信息"="", "流程参数"=""} ("data in"), "时间标识"=w500, "设备"=w492, "日志信息"="-->>启动成功") -> (w499:T2)
        n267 = call "总磷总氮操作日志.vi"("data in"=w499) -> ()  [unwired: 10 in, 1 out]
        n268 = call "Add State to Queue.vi"("State(s) In (\"\")"=w497) -> ("States Out"=w496:string)  [unwired: 14 in]
      }
      frame "Cal: Failure" {
        n269 = Get Date/Time In Seconds() -> (seconds since 1Jan1904=w507:timestamp)
        n270 = Bundle By Name(cluster=T2 {"时间标识"=timestamp(0 s since 1904-01-01), "设备"="", "日志信息"="", "流程参数"=""} ("data in"), "时间标识"=w507, "设备"=w502, "日志信息"="-->>启动失败") -> (w506:T2)
        n271 = call "总磷总氮操作日志.vi"("data in"=w506) -> ()  [unwired: 10 in, 1 out]
        n272 = call "Add State to Queue.vi"("State(s) In (\"\")"="exit" ("State(s) In (\"\")")) -> ("States Out"=w511:string)  [unwired: 14 in]
      }
      frame "Cal: Running" {
        n273 = global read "VAR总磷总氮全局变量.vi" "状态告警区"() -> (w523:T9)
        n274 = Less Or Equal?(x=w519, y=7200) -> (x <= y?=w517:bool)
        n275 = Unbundle By Name(w523) -> ("工作状态"=w524:u16)
        n276 = Select(t=w516, s=w517, f="exit") -> (s? t:f=w515:string)
        n277 = Equal?(x=w524, y=T5."空闲") -> (x = y?=w522:bool)
        n278 = Select(t="", s=w522, f=w515) -> (s? t:f=w520:string)
        n279 = call "Add State to Queue.vi"("State(s) In Front (\"\")"=w520, "State(s) In (\"\")"=w527) -> ("States Out"=w526:string)  [unwired: 13 in]
      }
      frame "Cal: Storing data" {
        n280 = case shown="1" w533 {
          tunnel: w536 -> [_ w538]
          frame 0, Default {
          }
          frame 1 {
            n281 = Get Date/Time In Seconds() -> (seconds since 1Jan1904=w542:timestamp)
            n282 = Bundle By Name(cluster=T2 {"时间标识"=timestamp(0 s since 1904-01-01), "设备"="", "日志信息"="", "流程参数"=""} ("data in"), "时间标识"=w542, "设备"=w538, "日志信息"="-->>存储数据") -> (w541:T2)
            n283 = call "总磷总氮操作日志.vi"("data in"=w541) -> ()  [unwired: 10 in, 1 out]
          }
        }
        n284 = Less Or Equal?(x=w533, y=60) -> (x <= y?=w531:bool)
        n285 = Select(t=w530, s=w531, f="") -> (s? t:f=w528:string)
        n286 = call "Add State to Queue.vi"("State(s) In Front (\"\")"=w528, "State(s) In (\"\")"=w535) -> ("States Out"=w534:string)  [unwired: 13 in]
      }
      frame "Cal: Finished" {
        n287 = case shown="1" w545 {
          tunnel: w544 -> [_ w551]
          tunnel: w543 -> [_ w550]
          frame 0, Default {
          }
          frame 1 {
            n288 = case shown="真" w550 {
              tunnel: ["测量结束>>" ("日志信息") "补测结束>>" ("日志信息")] -> w552
              frame False {
              }
              frame True {
              }
            }
            n289 = Get Date/Time In Seconds() -> (seconds since 1Jan1904=w555:timestamp)
            n290 = Bundle By Name(cluster=T2 {"时间标识"=timestamp(0 s since 1904-01-01), "设备"="", "日志信息"="", "流程参数"=""} ("data in"), "时间标识"=w555, "设备"=w551, "日志信息"=w552) -> (w554:T2)
            n291 = call "总磷总氮操作日志.vi"("data in"=w554) -> ()  [unwired: 10 in, 1 out]
          }
        }
        n292 = call "Add State to Queue.vi"("State(s) In (\"\")"=w549) -> ("States Out"=w548:string)  [unwired: 14 in]
      }
      frame "Cal: Next" {
      }
      frame "Cal: Wait restart" {
        n293 = local read "start"() -> (w565:timestamp)
        n294 = Get Date/Time In Seconds() -> (seconds since 1Jan1904=w566:timestamp)
        n295 = Subtract(x=w566, y=w565) -> (x-y=w564:dbl)
        n296 = Greater Or Equal?(x=w564, y=3600.0) -> (x >= y?=w568:bool)
        n297 = case shown="真" w568 {
          tunnel: ["Cal: Wait restart" ("State(s) In (\"\")") "Init: All\nInit: Process\nCal: Start\nCal: Running\nCal: Storing data\nCal: Finished\nCal: Next" ("State(s) In (\"\")")] -> w567
          frame False {
          }
          frame True {
            "重测" <- TRUE ("重测")
          }
        }
      }
      frame "exit", Default {
        n298 = Release Notifier(notifier=w581) -> ()  [unwired: 2 in, 3 out]
        n299 = Release Queue(queue=w582) -> ()  [unwired: 2 in, 3 out]
        n300 = Get Date/Time In Seconds() -> (seconds since 1Jan1904=w580:timestamp)
        n301 = Bundle By Name(cluster=T2 {"时间标识"=timestamp(0 s since 1904-01-01), "设备"="", "日志信息"="", "流程参数"=""} ("data in"), "时间标识"=w580, "设备"=w577, "日志信息"="流程结束>>") -> (w579:T2)
        n302 = call "总磷总氮操作日志.vi"("data in"=w579) -> ()  [unwired: 10 in, 1 out]
      }
    }
    n303 = feedback-in #1(w27) -> ()
    n304 = feedback #1() -> (w28:string)  [unwired: 1 in]
    n305 = Not Equal?(x=w28, y=w27) -> (x != y?=w26:bool)
    n306 = case shown="真" w26 {
      tunnel: w29 -> [_ w56]
      tunnel: w27 -> [_ w55]
      frame False {
      }
      frame True {
        n307 = Get Date/Time In Seconds() -> (seconds since 1Jan1904=w59:timestamp)
        n308 = Bundle By Name(cluster=T2 {"时间标识"=timestamp(0 s since 1904-01-01), "设备"="", "日志信息"="", "流程参数"=""} ("data in"), "时间标识"=w59, "设备"=w56, "日志信息"=w55) -> (w58:T2)
        n309 = call "总磷总氮操作日志.vi"("data in"=w58) -> ()  [unwired: 10 in, 1 out]
      }
    }
  }
